vi "checkin.vi"(8 "error in (no error)":errorcluster, 11 "GenericExperimentController in":refnum<class "GenericExperimentController.lvclass">) -> (0 "error out":errorcluster, 3 "GenericExperimentController out":refnum<class "GenericExperimentController.lvclass">)   [LabVIEW 2010, in "GenericExperimentController.lvclass"]
uses:
  GenericExperimentController.lvclass
  common/classes/GenericToplevelComponent/GenericToplevelComponent/GenericToplevelComponent.lvclass
  class_data.vi
  common/classes/GenericComponent/GenericComponent/GenericComponent.lvclass
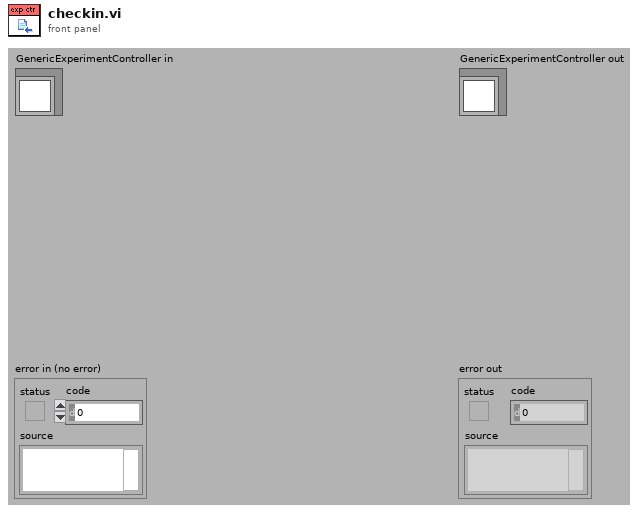
[diagram p1: front panel]
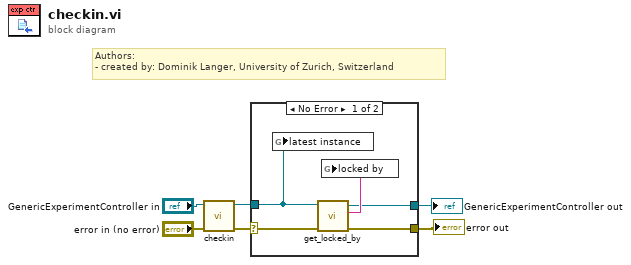
[diagram p0: block diagram]
diagram:
  # "Authors: \n- created by: Dominik Langer, University of Zurich, Switzerland"
  n1 = call-parent "checkin.vi"("error in (no error)"="error in (no error)", "GenericPlugin in"="GenericExperimentController in") -> ("error out"=w1:errorcluster, "GenericPlugin out"=w2:refnum<class "GenericExperimentController.lvclass">)  [unwired: 8 in]
  n2 = case shown="No Error" w1 {
    selector: w1 -> [w7 w13]
    tunnel: [w10 w13] -> w6
    tunnel: [w9 w12] -> w5
    tunnel: w2 -> [w8 w12]
    frame No Error {
      n3 = global write "class_data.vi" "latest instance"(w8) -> ()
      n4 = call "get_locked_by.vi"("error in (no error)"=w7, "GenericPlugin.lvclass in"=w8) -> ("error out"=w10:errorcluster, "locked by"=w11:string, "GenericPlugin.lvclass out"=w9:refnum<class "GenericExperimentController.lvclass">)  [unwired: 7 out]
      n5 = global write "class_data.vi" "locked by"(w11) -> ()
    }
    frame Error {
    }
  }
  "error out" <- w6
  "GenericExperimentController out" <- w5
